vi "Generate Type Descriptors.vi"(0 "Measurement Metadata":T1={"measurement_details"={"display_name"="Sample Streaming Measurement (.NET)", "version"="0.0.0.1"}, "measurement_signature"={"configuration_parameters_message_type"="ni.measurementlink.examples.SampleStreamingMeasurementConfigurations", "configuration_parameters"=[{"field_number"=1, "type"=enum."TYPE_STRING", "name"="name", "repeated"=FALSE, "annotations"=[], "message_type"=""}, {"field_number"=2, "type"=enum."TYPE_INT32", "name"="num_responses", "repeated"=FALSE, "annotations"=[], "message_type"=""}, {"field_number"=3, "type"=enum."TYPE_INT32", "name"="data_size", "repeated"=FALSE, "annotations"=[], "message_type"=""}, {"field_number"=4, "type"=enum."TYPE_BOOL", "name"="cumulative_data", "repeated"=FALSE, "annotations"=[], "message_type"=""}, {"field_number"=5, "type"=enum."TYPE_INT32", "name"="response_interval_in_ms", "repeated"=FALSE, "annotations"=[], "message_type"=""}, {"field_number"=6, "type"=enum."TYPE_INT32", "name"="error_on_index", "repeated"=FALSE, "annotations"=[], "message_type"=""}], "configuration_defaults"={"type_url"="type.googleapis.com/ni.measurementlink.examples.SampleStreamingMeasurementConfigurations", "value"=[10, 6, 60, 78, 97, 109, 101, 62, 16, 10, 24, 1, 32, 1, 40, 232, 7, 48, 255, 255, 255, 255, 255, 255, 255, 255, 255, 1]}, "outputs_message_type"="ni.measurementlink.examples.SampleStreamingMeasurementOutputs", "outputs"=[{"field_number"=1, "type"=enum."TYPE_STRING", "name"="name", "repeated"=FALSE, "annotations"=[], "message_type"=""}, {"field_number"=2, "type"=enum."TYPE_INT32", "name"="index", "repeated"=FALSE, "annotations"=[], "message_type"=""}, {"field_number"=3, "type"=enum."TYPE_INT32", "name"="data", "repeated"=TRUE, "annotations"=[], "message_type"=""}]}, "user_interface_details"=[{"file_url"="file:///C:/dev/ASW/Binaries/NetCore/Libraries/SampleStreamingMeasurement/Debug/SampleStreamingMeasurementWithGraph.measui"}, {"file_url"="file:///C:/dev/ASW/Binaries/NetCore/Libraries/SampleStreamingMeasurement/Debug/SampleStreamingMeasurementWithArrayIndicator.measui"}, {"file_url"="file:///C:/dev/ASW/Binaries/NetCore/Libraries/SampleStreamingMeasurement/Debug/SampleStreamingMeasurement.vi"}]}, 11 "error in (no error)":errorcluster) -> (4 "Configs Type":refnum<vi>, 6 "Configs typedef vi":refnum<vi>, 8 "Outputs Type":refnum<vi>, 10 "output Typedef VI":refnum<vi>, 15 "error out":errorcluster)   [LabVIEW 2021]
uses:
  Runtime/Clients/Measurement Service Client V2/RPC Messages/ni_measurementlink_measurement_v2_GetMetadataResponse.ctl
  Runtime/Clients/Measurement Service Client V2/RPC Messages/ni_measurementlink_measurement_v2_MeasurementDetails.ctl
  Runtime/Clients/Measurement Service Client V2/RPC Messages/ni_measurementlink_measurement_v2_MeasurementSignature.ctl
  Runtime/Clients/Measurement Service Client V2/RPC Messages/ni_measurementlink_measurement_v2_ConfigurationParameter.ctl
  Runtime/Clients/Measurement Service Client V2/RPC Messages/google_protobuf_Field_Kind.ctl
  Runtime/Clients/Measurement Service Client V2/RPC Messages/ni_measurementlink_measurement_v2_ConfigurationParameter_AnnotationsEntry.ctl
  Runtime/Clients/Measurement Service Client V2/RPC Messages/google_protobuf_Any.ctl
  Runtime/Clients/Measurement Service Client V2/RPC Messages/ni_measurementlink_measurement_v2_Output.ctl
  Runtime/Clients/Measurement Service Client V2/RPC Messages/ni_measurementlink_measurement_v2_Output_AnnotationsEntry.ctl
  Runtime/Clients/Measurement Service Client V2/RPC Messages/ni_measurementlink_measurement_v2_UserInterfaceDetails.ctl
  Runtime/Clients/Measurement Service Client V2/Measurement Service Client V2.lvlib
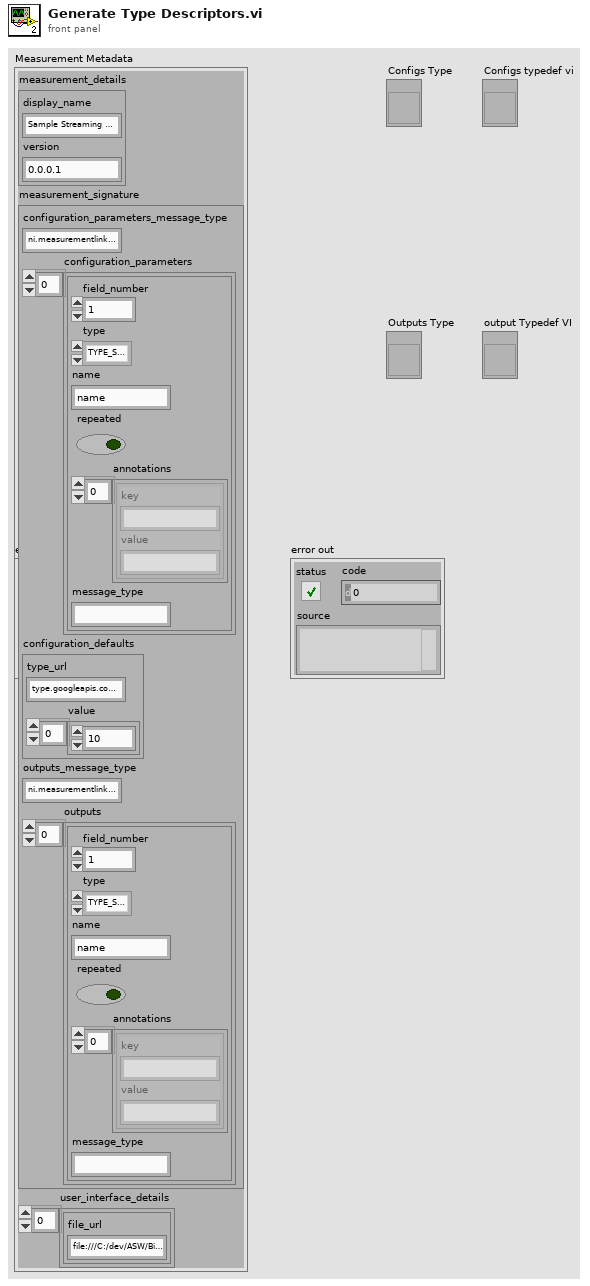
[diagram p1: front panel]
types:
  T1 = typedef "Measurement Service Client V2.lvlib/ni_measurementlink_measurement_v2_GetMetadataResponse.ctl" = cluster{"measurement_details":T2, "measurement_signature":T3, "user_interface_details":T10[]}
  T2 = typedef "Measurement Service Client V2.lvlib/ni_measurementlink_measurement_v2_MeasurementDetails.ctl" = cluster{"display_name":string, "version":string}
  T3 = typedef "Measurement Service Client V2.lvlib/ni_measurementlink_measurement_v2_MeasurementSignature.ctl" = cluster{"configuration_parameters_message_type":string, "configuration_parameters":T4[], "configuration_defaults":T7, "outputs_message_type":string, "outputs":T8[]}
  T4 = typedef "Measurement Service Client V2.lvlib/ni_measurementlink_measurement_v2_ConfigurationParameter.ctl" = cluster{"field_number":i32, "type":T5, "name":string, "repeated":bool, "annotations":T6[], "message_type":string}
  T5 = typedef "Measurement Service Client V2.lvlib/google_protobuf_Field_Kind.ctl" = enum32{"TYPE_UNKNOWN", "TYPE_DOUBLE", "TYPE_FLOAT", "TYPE_INT64", "TYPE_UINT64", "TYPE_INT32", "TYPE_FIXED64", "TYPE_FIXED32", "TYPE_BOOL", "TYPE_STRING", "TYPE_GROUP", "TYPE_MESSAGE", "TYPE_BYTES", "TYPE_UINT32", "TYPE_ENUM", "TYPE_SFIXED32", "TYPE_SFIXED64", "TYPE_SINT32", "TYPE_SINT64"}
  T6 = typedef "Measurement Service Client V2.lvlib/ni_measurementlink_measurement_v2_ConfigurationParameter_AnnotationsEntry.ctl" = cluster{"key":string, "value":string}
  T7 = typedef "Measurement Service Client V2.lvlib/google_protobuf_Any.ctl" = cluster{"type_url":string, "value":u8[]}
  T8 = typedef "Measurement Service Client V2.lvlib/ni_measurementlink_measurement_v2_Output.ctl" = cluster{"field_number":i32, "type":T5, "name":string, "repeated":bool, "annotations":T9[], "message_type":string}
  T9 = typedef "Measurement Service Client V2.lvlib/ni_measurementlink_measurement_v2_Output_AnnotationsEntry.ctl" = cluster{"key":string, "value":string}
  T10 = typedef "Measurement Service Client V2.lvlib/ni_measurementlink_measurement_v2_UserInterfaceDetails.ctl" = cluster{"file_url":string}
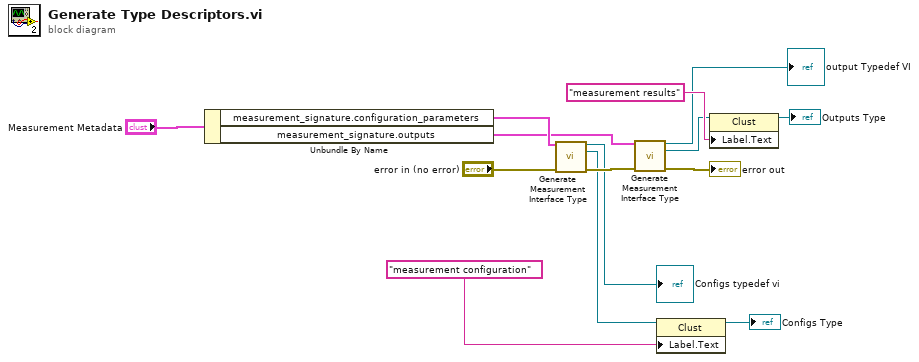
[diagram p0: block diagram]
diagram:
  n1 = Unbundle By Name("Measurement Metadata") -> ("measurement_signature.configuration_parameters"=w12:T4[], "measurement_signature.outputs"=w11:T8[])
  n2 = call "Generate Measurement Interface Type.vi"("Parameters"=w12, "error in (no error)"="error in (no error)") -> ("VI out"=→"Configs typedef vi":refnum<vi>, "Clust Refnum"=w8:refnum<vi>, "error out"=w10:errorcluster)  [unwired: 10 in, 1 out]
  n3 = call "Generate Measurement Interface Type.vi"("Parameters"=w11, "error in (no error)"=w10) -> ("VI out"=→"output Typedef VI":refnum<vi>, "Clust Refnum"=w4:refnum<vi>, "error out"=→"error out":errorcluster)  [unwired: 10 in, 1 out]
  n4 = property class="Clust"(reference=w8, "Label.Text"="measurement configuration") -> (reference out=→"Configs Type":refnum<vi>)  [unwired: 1 in, 1 out]
  n5 = property class="Clust"(reference=w4, "Label.Text"="measurement results") -> (reference out=→"Outputs Type":refnum<vi>)  [unwired: 1 in, 1 out]
